vi "Send Register Settings Changes.vi"(7 "Message Priority (Normal)":T2=enum."Normal", 8 "error in (no error)":errorcluster, 10 "Settings Data":T1, 11 "Message Enqueuer":refnum<class "Message Enqueuer.lvclass">) -> (0 "error out":errorcluster, 3 "Message Enqueuer out":refnum<class "Message Enqueuer.lvclass">)   [LabVIEW 2015, in "VI App Store.lvlib" / "Register Settings Changes Msg.lvclass"]
doc: "This VI sends the message to an actor."
uses:
  Register Settings Changes Msg.lvclass
  <vilib>/ActorFramework/Message Enqueuer/Message Enqueuer.lvclass
  <vilib>/ActorFramework/Message Enqueuer/Message Priority.ctl
  Classes/Settings Item/Settings Data.ctl
  Register Settings Changes Msg.lvclass/Register Settings Changes Msg.ctl
  <vilib>/ActorFramework/Message Enqueuer/Message Enqueuer.lvclass/Message Enqueuer.ctl
  <vilib>/ActorFramework/Message Priority Queue/Priority Enqueue.vi
  Classes/Settings Item/Settings.lvclass
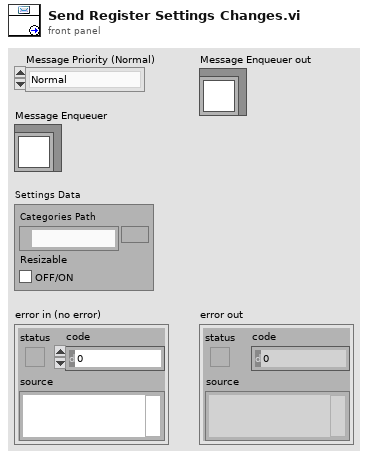
[diagram p1: front panel]
types:
  T1 = typedef "Item Actor.lvlib/Settings.lvclass/Settings Data.ctl" = cluster{"Categories Path":path, "Resizable":bool}
  T2 = typedef "Actor Framework.lvlib/Message Enqueuer.lvclass/Message Priority.ctl" = enum16{"Low", "Normal", "High"}
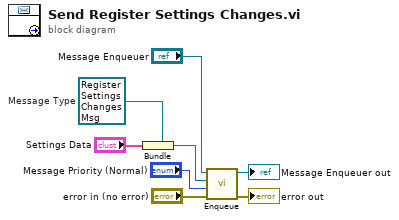
[diagram p0: block diagram]
diagram:
  w2 = refnum<class "Register Settings Changes Msg.lvclass"> refnum  # Message Type
  n1 = Bundle(cluster=w2, "Settings Data") -> (w3:refnum<class "Register Settings Changes Msg.lvclass">)
  n2 = call <vilib>:"Enqueue.vi"("error in (no error)"="error in (no error)", "Message Priority (Normal)"="Message Priority (Normal)", "Message"=w3, "Message Enqueuer in"="Message Enqueuer") -> ("error out"=→"error out":errorcluster, "Message Enqueuer out"=→"Message Enqueuer out":refnum<class "Message Enqueuer.lvclass">)  [unwired: 6 in]
